vi "AUTON_Index.vi"(0 "Auton Array":dbl[][](array[numeric]), 5 "MeasuredHeading":dbl, 7 "LeftEncoder":dbl, 9 "RightEncoder":dbl) -> (4 "Left Drive":dbl, 6 "Right Drive":dbl, 8 "Indexer":dbl, 10 "Shooter Elevation":dbl, 13 "Flipper":dbl, 14 "Roller":dbl, 15 "Shooter Wheels":dbl)   [LabVIEW 2012]
uses:
  Robot Global Data.vi
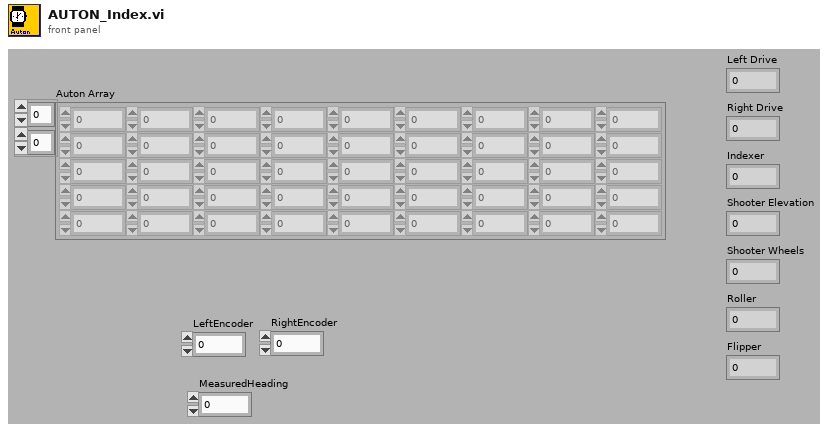
[diagram p1: front panel]
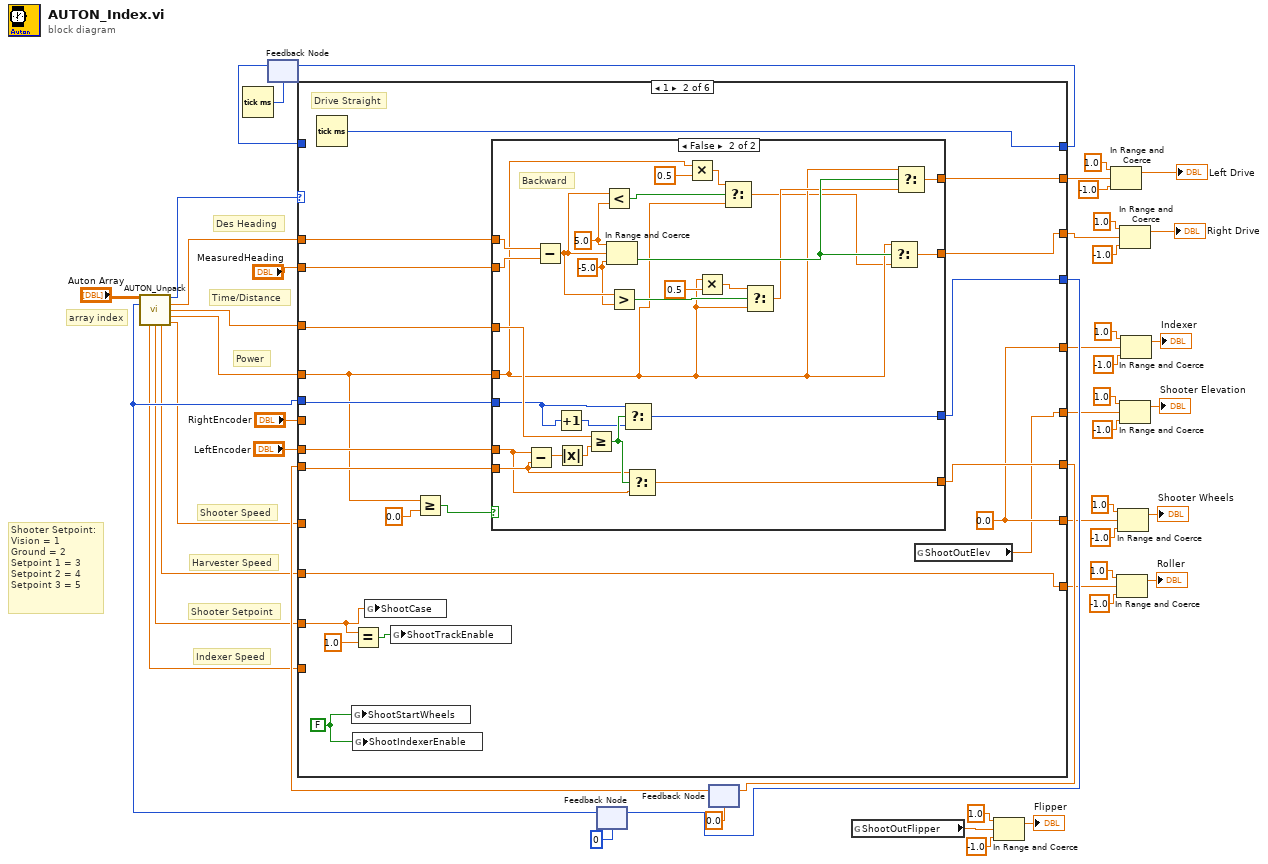
[diagram p0: block diagram]
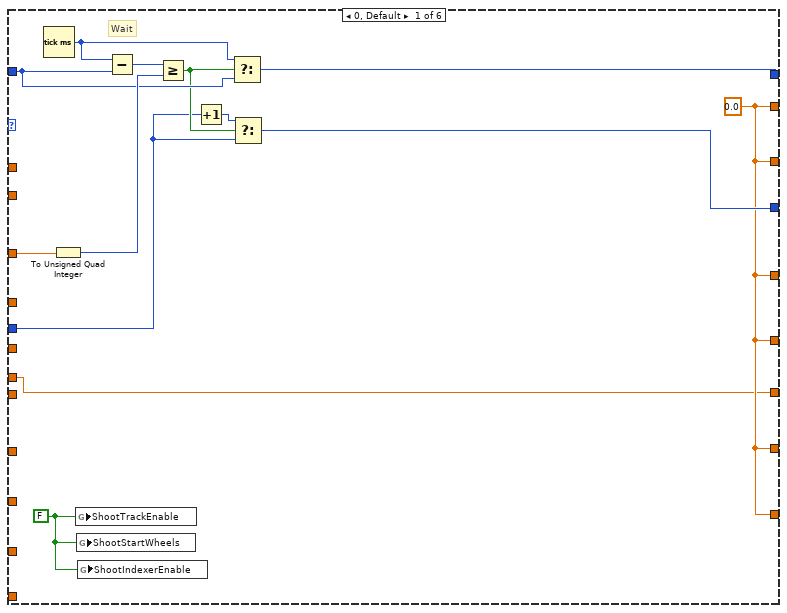
[diagram p2: hidden frame]
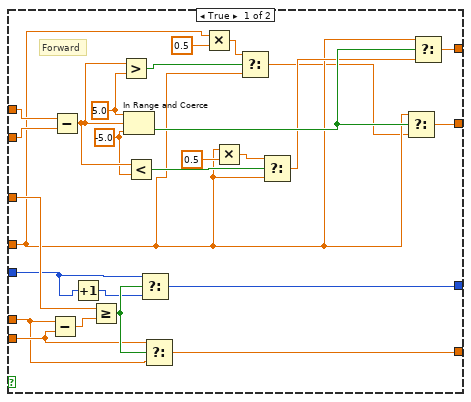
[diagram p3: hidden frame]
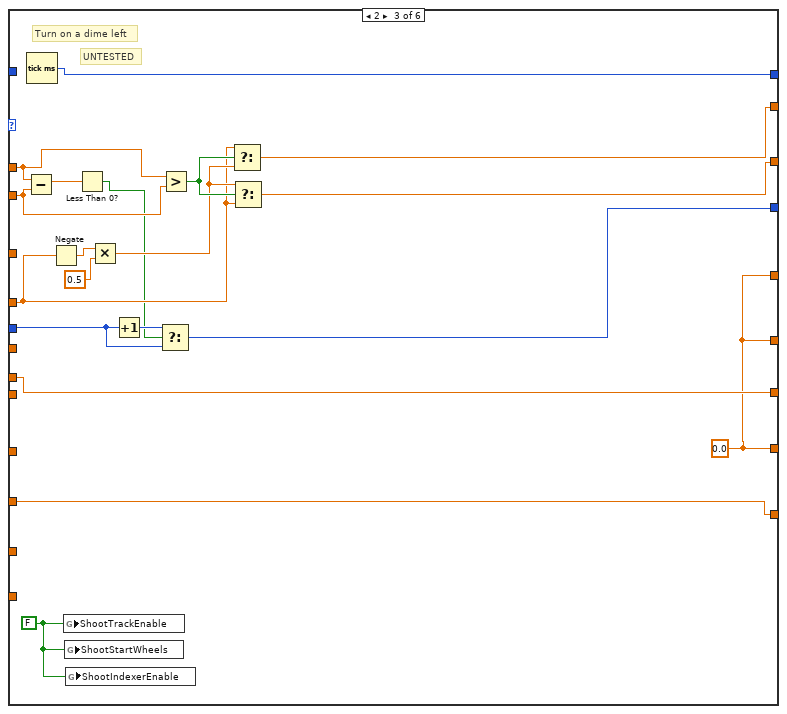
[diagram p4: hidden frame]
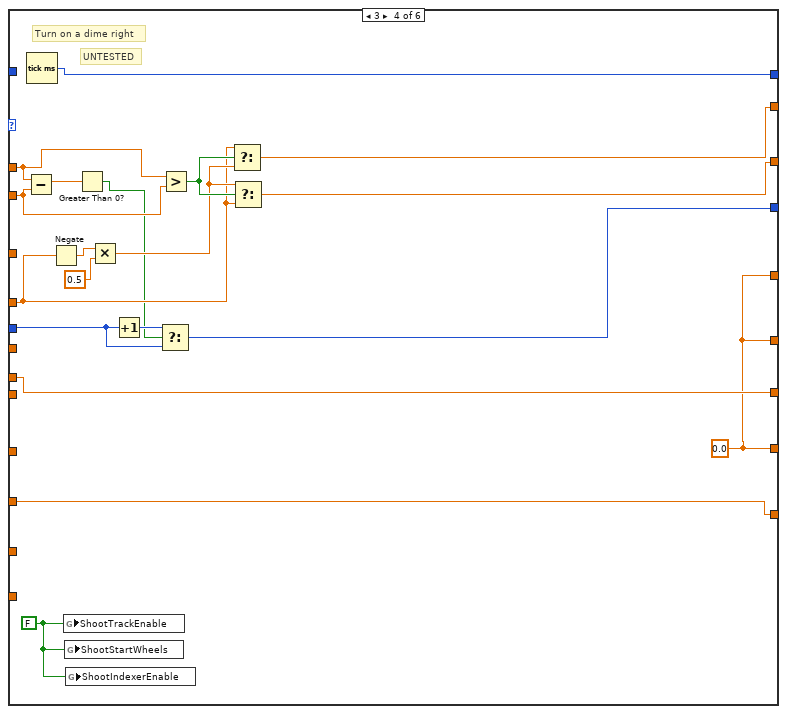
[diagram p5: hidden frame]
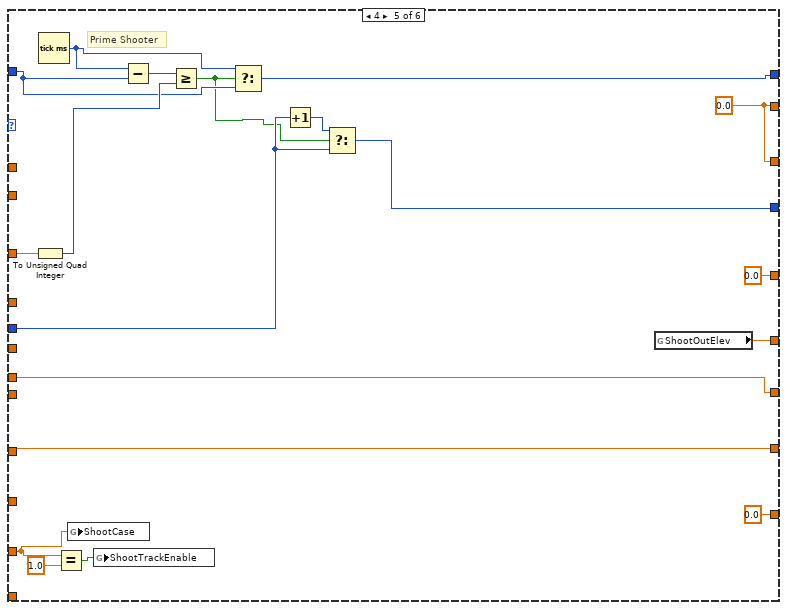
[diagram p6: hidden frame]
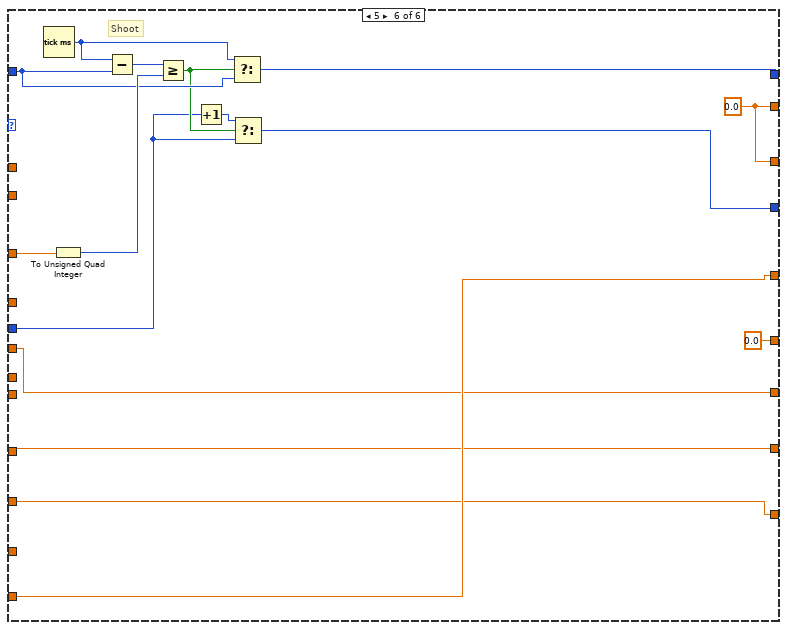
[diagram p7: hidden frame]
diagram:
  # "Shooter Setpoint:\nVision = 1\nGround = 2\nSetpoint 1 = 3\nSetpoint 2 = 4\nSetpoint 3 = 5"
  # "Indexer Speed"
  # "Shooter Speed"
  # "Shooter Setpoint"
  # "Harvester Speed"
  # "Des Heading"
  # "Time/Distance"
  # "Power"
  # "array index"
  n1 = Tick Count (ms)() -> (millisecond timer value=w46:u32)
  n2 = feedback #1(w46) -> (w48:u32)
  n3 = feedback #2(0) -> (w25:i32)
  n4 = call "AUTON_Unpack.vi"("all rows"="Auton Array", "Index"=w25) -> ("Primitive ID"=w29:i16, "Desired Heading"=w27:dbl, "Time/Distance"=w26:dbl, "Power"=w28:dbl, "Indexer Speed"=w21:dbl, "Shooter Setpoint"=w22:dbl, "Harvester Speed"=w23:dbl, "Shooter Speed"=w24:dbl)  [unwired: 6 in]
  n5 = feedback #3(0.0) -> (w31:dbl)
  n6 = case shown="1" w29 {
    tunnel: [w54 w81 w150 w169 w188 w201] -> w34
    tunnel: w25 -> [w55 w76 w153 w172 w179 w202]
    tunnel: [w62 w73 w155 w174 w177 w209] -> w36
    tunnel: w48 -> [w59 _ _ _ w178 w206]
    tunnel: w26 -> [w53 w82 _ _ w180 w200]
    tunnel: w27 -> [_ w80 w148 w167 _ _]
    tunnel: [w52 w78 w151 w170 w193 w199] -> w44
    tunnel: [w52 w77 w152 w171 w193 w199] -> w37
    tunnel: w28 -> [_ w72 w142 w161 _ _]
    tunnel: "LeftEncoder" -> [w50 w74 w149 w168 w192 _]
    tunnel: "MeasuredHeading" -> [_ w79 w147 w166 _ _]
    tunnel: "RightEncoder" -> [_ _ _ _ _ w194]
    tunnel: w31 -> [_ w75 _ _ _ _]
    tunnel: [w50 w83 w149 w168 w192 w194] -> w30
    tunnel: w24 -> [_ _ _ _ w191 w196]
    tunnel: w23 -> [_ w67 w139 w158 _ w195]
    tunnel: w22 -> [_ w64 _ _ w184 _]
    tunnel: w21 -> [_ _ _ _ _ w198]
    tunnel: [w52 w67 w139 w158 0.0 ("Harvester Speed") w195] -> w5
    tunnel: [w52 w69 w140 w159 w191 w196] -> w4
    tunnel: [w52 w63 w140 w159 w176 0.0 ("ShootOutElev")] -> w3
    tunnel: [w52 w69 w140 w159 0.0 ("Numeric") w198] -> w2
    frame 0, Default {
      w51 = FALSE ("ShootTrackEnable")
      w52 = 0.0 ("Numeric")
      # "Wait"
      n7 = Tick Count (ms)() -> (millisecond timer value=w58:u32)
      n8 = To Unsigned Quad Integer(1:w53) -> (0:w60:u64)
      n9 = global write "Robot Global Data.vi" "ShootTrackEnable"(w51) -> ()
      n10 = global write "Robot Global Data.vi" "ShootStartWheels"(w51) -> ()
      n11 = global write "Robot Global Data.vi" "ShootIndexerEnable"(w51) -> ()
      n12 = Subtract(x=w58, y=w59) -> (x-y=w61:u32)
      n13 = Greater Or Equal?(x=w61, y=w60) -> (x >= y?=w57:bool)
      n14 = Increment(x=w55) -> (x+1=w56:i32)
      n15 = Select(t=w58, s=w57, f=w59) -> (s? t:f=w62:u32)
      n16 = Select(t=w56, s=w57, f=w55) -> (s? t:f=w54:i32)
    }
    frame 1 {
      w68 = FALSE ("ShootTrackEnable")
      w69 = 0.0 ("Numeric")
      # "Drive Straight"
      n17 = Tick Count (ms)() -> (millisecond timer value=w73:u32)
      n18 = global write "Robot Global Data.vi" "ShootStartWheels"(w68) -> ()
      n19 = Equal?(x=w64, y=1.0) -> (x = y?=w65:bool)
      n20 = global write "Robot Global Data.vi" "ShootIndexerEnable"(w68) -> ()
      n21 = global write "Robot Global Data.vi" "ShootCase"(w64) -> ()
      n22 = global write "Robot Global Data.vi" "ShootTrackEnable"(w65) -> ()
      n23 = Greater Or Equal?(x=w72, y=0.0) -> (x >= y?=w70:bool)
      n24 = case shown="False" w70 {
        tunnel: [w109 w136] -> w83
        tunnel: w82 -> [w107 w135]
        tunnel: [w105 w133] -> w81
        tunnel: w80 -> [w104 w132]
        tunnel: w79 -> [w103 w131]
        tunnel: [w101 w129] -> w78
        tunnel: [w100 w128] -> w77
        tunnel: w72 -> [w89 w117]
        tunnel: w76 -> [w86 w114]
        tunnel: w75 -> [w85 w113]
        tunnel: w74 -> [w84 w112]
        frame True {
          w97 = -5.0 ("lower limit")
          w99 = 5.0 ("upper limit")
          # "Forward"
          n25 = Subtract(x=w84, y=w85) -> (x-y=w108:dbl)
          n26 = Subtract(x=w104, y=w103) -> (x-y=w98:dbl)
          n27 = Increment(x=w86) -> (x+1=w87:i32)
          n28 = Greater Or Equal?(x=w107, y=w108) -> (x >= y?=w106:bool)
          n29 = Greater?(x=w98, y=w99) -> (0:w92:bool)
          n30 = In Range and Coerce(upper limit=w99, x=w98, lower limit=w97) -> (In Range?=w102:bool)  [unwired: 1 out]
          n31 = Less?(x=w98, y=w97) -> (x < y?=w96:bool)
          n32 = Select(t=w86, s=w106, f=w87) -> (s? t:f=w105:i32)
          n33 = Select(t=w85, s=w106, f=w84) -> (s? t:f=w109:dbl)
          n34 = Multiply(x=w89, y=0.5) -> (x*y=w91:dbl)
          n35 = Multiply(x=w89, y=0.5) -> (x*y=w94:dbl)
          n36 = Select(t=w91, s=w92, f=w89) -> (s? t:f=w88:dbl)
          n37 = Select(t=w94, s=w96, f=w89) -> (s? t:f=w93:dbl)
          n38 = Select(t=w89, s=w102, f=w88) -> (s? t:f=w100:dbl)
          n39 = Select(t=w89, s=w102, f=w93) -> (s? t:f=w101:dbl)
        }
        frame False {
          w125 = -5.0 ("lower limit")
          w127 = 5.0 ("upper limit")
          # "Backward"
          n40 = Subtract(x=w112, y=w113) -> (x-y=w110:dbl)
          n41 = Subtract(x=w132, y=w131) -> (x-y=w126:dbl)
          n42 = Increment(x=w114) -> (x+1=w115:i32)
          n43 = Absolute Value(x=w110) -> (abs(x)=w111:dbl)
          n44 = Greater Or Equal?(x=w135, y=w111) -> (x >= y?=w134:bool)
          n45 = Less?(x=w126, y=w127) -> (x < y?=w120:bool)
          n46 = In Range and Coerce(upper limit=w127, x=w126, lower limit=w125) -> (In Range?=w130:bool)  [unwired: 1 out]
          n47 = Greater?(x=w126, y=w125) -> (0:w124:bool)
          n48 = Select(t=w114, s=w134, f=w115) -> (s? t:f=w133:i32)
          n49 = Select(t=w113, s=w134, f=w112) -> (s? t:f=w136:dbl)
          n50 = Multiply(x=w117, y=0.5) -> (x*y=w119:dbl)
          n51 = Multiply(x=w117, y=0.5) -> (x*y=w122:dbl)
          n52 = Select(t=w119, s=w120, f=w117) -> (s? t:f=w116:dbl)
          n53 = Select(t=w122, s=w124, f=w117) -> (s? t:f=w121:dbl)
          n54 = Select(t=w117, s=w130, f=w116) -> (s? t:f=w128:dbl)
          n55 = Select(t=w117, s=w130, f=w121) -> (s? t:f=w129:dbl)
        }
      }
      n56 = global read "Robot Global Data.vi" "ShootOutElev"() -> (w63:dbl)
    }
    frame 2 {
      w140 = 0.0 ("Numeric")
      w141 = FALSE ("ShootTrackEnable")
      # "UNTESTED"
      # "Turn on a dime left"
      n57 = Subtract(x=w148, y=w147) -> (x-y=w138:dbl)
      n58 = Tick Count (ms)() -> (millisecond timer value=w155:u32)
      n59 = Negate(x=w142) -> (-x=w145:dbl)
      n60 = global write "Robot Global Data.vi" "ShootTrackEnable"(w141) -> ()
      n61 = global write "Robot Global Data.vi" "ShootStartWheels"(w141) -> ()
      n62 = global write "Robot Global Data.vi" "ShootIndexerEnable"(w141) -> ()
      n63 = Less Than 0?(x=w138) -> (x < 0?=w137:bool)
      n64 = Multiply(x=w145, y=0.5) -> (x*y=w143:dbl)
      n65 = Increment(x=w153) -> (x+1=w154:i32)
      n66 = Select(t=w154, s=w137, f=w153) -> (s? t:f=w150:i32)
      n67 = Greater?(x=w148, y=w147) -> (0:w146:bool)
      n68 = Select(t=w142, s=w146, f=w143) -> (s? t:f=w151:dbl)
      n69 = Select(t=w143, s=w146, f=w142) -> (s? t:f=w152:dbl)
    }
    frame 3 {
      w159 = 0.0 ("Numeric")
      w160 = FALSE ("ShootTrackEnable")
      # "UNTESTED"
      # "Turn on a dime right"
      n70 = Subtract(x=w167, y=w166) -> (x-y=w157:dbl)
      n71 = Tick Count (ms)() -> (millisecond timer value=w174:u32)
      n72 = Negate(x=w161) -> (-x=w164:dbl)
      n73 = global write "Robot Global Data.vi" "ShootTrackEnable"(w160) -> ()
      n74 = global write "Robot Global Data.vi" "ShootStartWheels"(w160) -> ()
      n75 = global write "Robot Global Data.vi" "ShootIndexerEnable"(w160) -> ()
      n76 = Greater Than 0?(x=w157) -> (x > 0?=w156:bool)
      n77 = Multiply(x=w164, y=0.5) -> (x*y=w162:dbl)
      n78 = Increment(x=w172) -> (x+1=w173:i32)
      n79 = Select(t=w173, s=w156, f=w172) -> (s? t:f=w169:i32)
      n80 = Greater?(x=w167, y=w166) -> (0:w165:bool)
      n81 = Select(t=w161, s=w165, f=w162) -> (s? t:f=w170:dbl)
      n82 = Select(t=w162, s=w165, f=w161) -> (s? t:f=w171:dbl)
    }
    frame 4 {
      w193 = 0.0 ("Power")
      # "Prime Shooter"
      n83 = To Unsigned Quad Integer(1:w180) -> (0:w182:u64)
      n84 = Tick Count (ms)() -> (millisecond timer value=w181:u32)
      n85 = Equal?(x=w184, y=1.0) -> (x = y?=w185:bool)
      n86 = global write "Robot Global Data.vi" "ShootCase"(w184) -> ()
      n87 = global write "Robot Global Data.vi" "ShootTrackEnable"(w185) -> ()
      n88 = Subtract(x=w181, y=w178) -> (x-y=w183:u32)
      n89 = Greater Or Equal?(x=w183, y=w182) -> (x >= y?=w175:bool)
      n90 = Select(t=w181, s=w175, f=w178) -> (s? t:f=w177:u32)
      n91 = Increment(x=w179) -> (x+1=w187:i32)
      n92 = Select(t=w187, s=w175, f=w179) -> (s? t:f=w188:i32)
      n93 = global read "Robot Global Data.vi" "ShootOutElev"() -> (w176:dbl)
    }
    frame 5 {
      w199 = 0.0 ("Numeric")
      # "Shoot"
      n94 = Tick Count (ms)() -> (millisecond timer value=w205:u32)
      n95 = To Unsigned Quad Integer(1:w200) -> (0:w207:u64)
      n96 = Subtract(x=w205, y=w206) -> (x-y=w208:u32)
      n97 = Greater Or Equal?(x=w208, y=w207) -> (x >= y?=w204:bool)
      n98 = Increment(x=w202) -> (x+1=w203:i32)
      n99 = Select(t=w205, s=w204, f=w206) -> (s? t:f=w209:u32)
      n100 = Select(t=w203, s=w204, f=w202) -> (s? t:f=w201:i32)
    }
  }
  n101 = feedback-in #1(w36) -> ()
  n102 = feedback-in #2(w34) -> ()
  n103 = feedback-in #3(w30) -> ()
  n104 = global read "Robot Global Data.vi" "ShootOutFlipper"() -> (w1:dbl)
  n105 = In Range and Coerce(upper limit=1.0, x=w1, lower limit=-1.0) -> (coerced(x)=→"Flipper":dbl)  [unwired: 1 out]
  n106 = In Range and Coerce(upper limit=1.0, x=w44, lower limit=-1.0) -> (coerced(x)=→"Left Drive":dbl)  [unwired: 1 out]
  n107 = In Range and Coerce(upper limit=1.0, x=w5, lower limit=-1.0) -> (coerced(x)=→"Roller":dbl)  [unwired: 1 out]
  n108 = In Range and Coerce(upper limit=1.0, x=w4, lower limit=-1.0) -> (coerced(x)=→"Shooter Wheels":dbl)  [unwired: 1 out]
  n109 = In Range and Coerce(upper limit=1.0, x=w37, lower limit=-1.0) -> (coerced(x)=→"Right Drive":dbl)  [unwired: 1 out]
  n110 = In Range and Coerce(upper limit=1.0, x=w3, lower limit=-1.0) -> (coerced(x)=→"Shooter Elevation":dbl)  [unwired: 1 out]
  n111 = In Range and Coerce(upper limit=1.0, x=w2, lower limit=-1.0) -> (coerced(x)=→"Indexer":dbl)  [unwired: 1 out]
